vi "ILS_LV.vi"() -> ()   [LabVIEW 2013]
panel:
  out "result":dbl
  in  "n2":dbl
  in  "n1":dbl
  # "ILS"
  # "MODIFICADOOOOOOOOOOOOOOOOOOOOO"
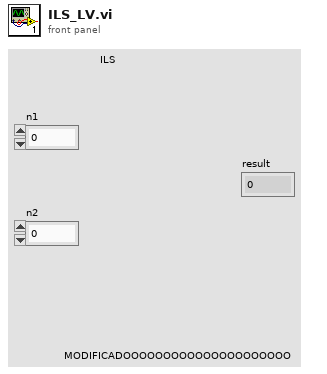
[diagram p1: front panel]
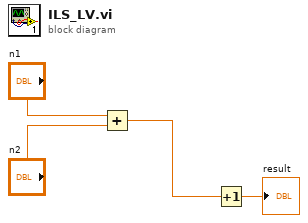
[diagram p0: block diagram]
diagram:
  n1 = Add(x="n1", y="n2") -> (x+y=w2:dbl)
  n2 = Increment(x=w2) -> (x+1=→"result":dbl)
